vi "Custom.vi"(11 "General settings":T1) -> (2 "Vortex":dbl[][](array[numeric]))   [LabVIEW 2018]
uses:
  Controls/General Setting.ctl
  Controls/Buttons/Running Button.ctl
panel:
  in  "weight":dbl
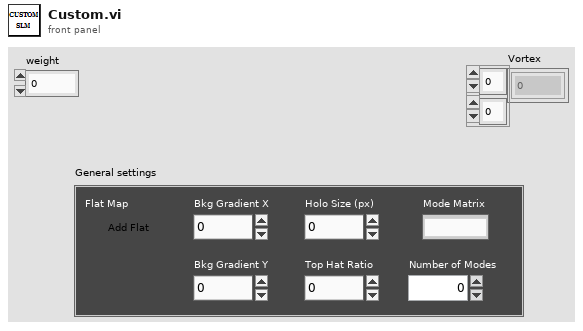
[diagram p1: front panel]
types:
  T1 = typedef "General Setting.ctl" = cluster{"Flat Map":T2, "Bkg Gradient X":dbl, "Bkg Gradient Y":dbl, "Holo Size (px)":i32, "Top Hat Ratio":dbl, "Number of Modes":i8, "Mode Matrix":u16}
  T2 = typedef "Running Button.ctl" = bool
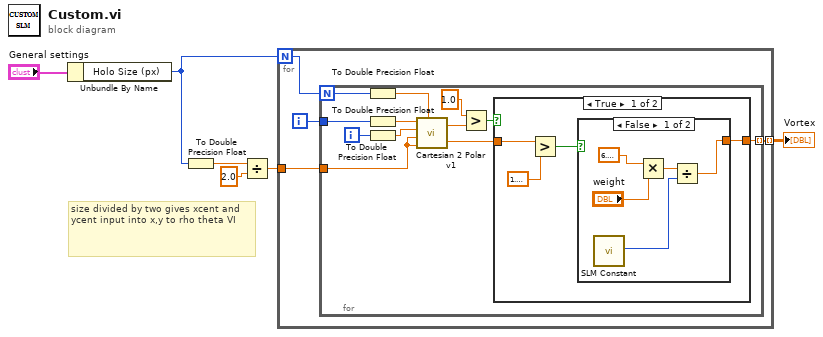
[diagram p0: block diagram]
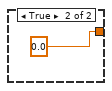
[diagram p2: hidden frame]
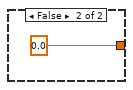
[diagram p3: hidden frame]
diagram:
  # "size divided by two gives xcent and ycent input into x,y to rho theta VI"
  n1 = Unbundle By Name("General settings") -> ("Holo Size (px)"=w3:i32)
  n2 = To Double Precision Float(number=w3) -> (double precision float=w2:dbl)
  n3 = Divide(x=w2, y=2.0) -> (x/y=w6:dbl)
  n4 = for {
    N: w3 -> [w7]
    tunnel: [w9] -> w1 mode=indexing
    tunnel: w6 -> [w8]
    i -> [w10]
    n5 = for {
      N: w7 -> [w16]
      tunnel: w10 -> [w21]
      tunnel: [w15] -> w9 mode=indexing
      tunnel: w8 -> [w17]
      i -> [w22]
      n6 = To Double Precision Float(number=w16) -> (double precision float=w14:dbl)
      n7 = To Double Precision Float(number=w21) -> (double precision float=w13:dbl)
      n8 = To Double Precision Float(number=w22) -> (double precision float=w12:dbl)
      n9 = call "Cartesian 2 Polar v1.vi"("x"=w13, "y"=w12, "xcent"=w17, "ycent"=w17, "diam"=w14) -> ("rho"=w19:dbl, "theta"=w11:dbl)
      n10 = Greater?(x=1.0, y=w19) -> (0:w20:bool)
      n11 = case shown="True" w20 {
        tunnel: w11 -> [w26 _]
        tunnel: [w23 0.0 ("zernike")] -> w15
        frame True {
          n12 = Greater?(x=w26, y=1.5707963267948966) -> (0:w24:bool)
          n13 = case shown="False" w24 {
            tunnel: [w27 0.0] -> w23
            frame False {
              n14 = call "SLM Constant.vi"() -> ("Gray Level Corresponding to 2Pi"=w28:i32)  [unwired: 10 in, 9 out]
              n15 = Multiply(x=6.283185307179586, y="weight") -> (x*y=w29:dbl)
              n16 = Divide(x=w29, y=w28) -> (x/y=w27:dbl)
            }
            frame True {
            }
          }
        }
        frame False {
        }
      }
    }
  }
  "Vortex" <- w1
